vi "GlobalVarsNetwork.vi"() -> ()   [LabVIEW 2023]
panel:
  in  "Network Vars":T1={"XY_IP_ADDRESS"="192.168.10.11", "Z_IP_ADDRESS"="192.168.10.12", "Port"=4000, "connection refnum x,y"=refnum, "connection refnum z"=refnum}
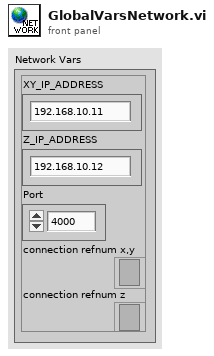
[diagram p1: front panel]
types:
  T1 = cluster{"XY_IP_ADDRESS":string, "Z_IP_ADDRESS":string, "Port":u16, "connection refnum x,y":refnum<k5>, "connection refnum z":refnum<k5>}
diagram:
